vi "Read Timeout.vi"(8 "error in (no error)":errorcluster, 11 "bt_Synch in":refnum<class "bt_WaitOn_Synch.lvclass">) -> (0 "error out":errorcluster, 2 "Timeout":i32=-1, 3 "bt_Synch out":refnum<class "bt_WaitOn_Synch.lvclass">)   [LabVIEW 2021, in "BT.lvlib" / "bt_WaitOn_Synch.lvclass"]
uses:
  bt_WaitOn_Synch.lvclass
  bt_WaitOn_Synch.lvclass/bt_WaitOn_Synch.ctl
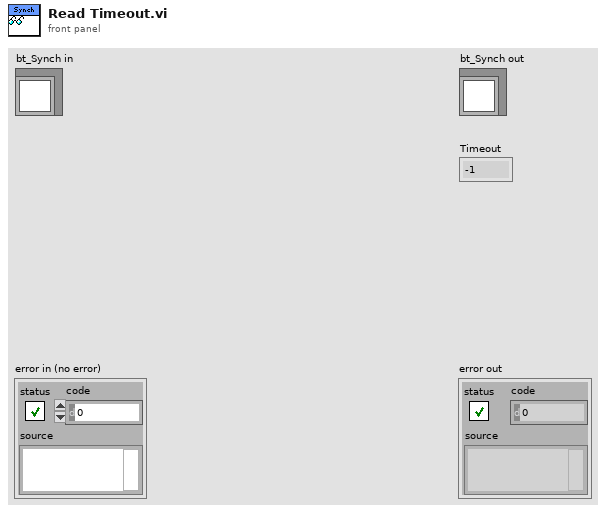
[diagram p1: front panel]
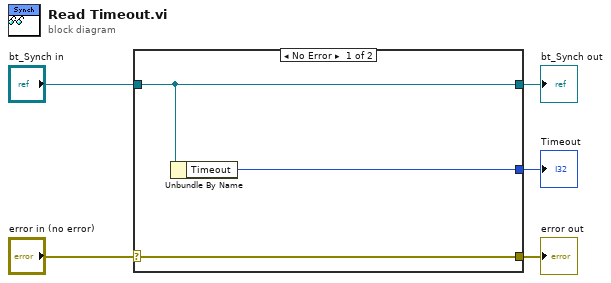
[diagram p0: block diagram]
diagram:
  n1 = case shown="No Error" "error in (no error)" {
    selector: "error in (no error)" -> [w8 w9]
    tunnel: [w8 w9] -> w4
    tunnel: [w7 w10] -> w2
    tunnel: "bt_Synch in" -> [w7 w10]
    tunnel: [w6 _] -> w1
    frame No Error {
      n2 = Unbundle By Name(w7) -> ("Timeout"=w6:i32)
    }
    frame Error {
    }
  }
  "error out" <- w4
  "bt_Synch out" <- w2
  "Timeout" <- w1
